vi "BigSky-Sandbox.vi"() -> ()   [LabVIEW 2018]
doc: "This example performs a serial port write and a serial port read. The parameters set for the serial port must match the parameters of the connected instrument or device. The VISA Configure Serial Port VI sets the configuration parameters. The front panel displays the controls used to configure the basic parameters, such as baud rate, data bits, and parity. The VI passes the VISA resource name to other VIs that perform operations on that VISA resource. The VISA Write function sends a command to the serial device and the VISA Read function returns data based on the command. The VISA Close function then closes the reference to the serial device. It is important to close the reference; otherwise, further communication through that port might not be possible."
uses:
  Program Files/National Instruments/LabVIEW 2018/examples/Instrument IO/Serial/support/Serial - Settings.ctl
  <vilib>/Instr/_visa.llb/VISA Configure Serial Port (Instr).vi
panel:
  out "read buffer":string
  in  "write buffer 2":string
  out "Write return count":u32
  in  "byte count":u32=1024
  in  "write buffer":string
  out "Read return count":u32
  in  "Serial Settings":T1={"baud rate"=9600, "data bits"=8, "parity"=enum."None", "stop bits"=10, "flow control"=0} {"flow control" items=["None"=0, "XON/XOFF"=1, "RTS/CTS"=2, "DTR/DSR"=4]; "stop bits" items=["1.0"=10, "1.5"=15, "2.0"=20]; "data bits" min=5 max=8 step=1; "baud rate" items=["75"=75, "110"=110, "134"=134, "150"=150, "300"=300, "600"=600, "1200"=1200, "1800"=1800, "2400"=2400, "4800"=4800, "7200"=7200, "9600"=9600, "14400"=14400, "19200"=19200, "28800"=28800, "38400"=38400, "56000"=56000, "57600"=57600, "115200"=115200, "128000"=128000, "230400"=230400]}
  in  "delay before read (ms)":u32=500
  out "Response":string
  in  "VISA resource name":refnum<visa-resource-name>="COM1"
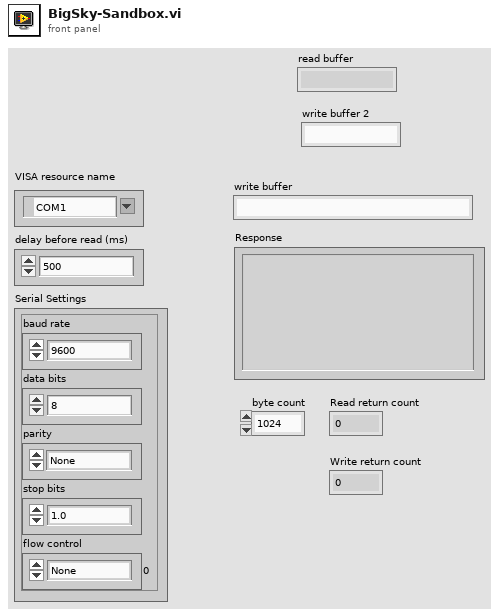
[diagram p1: front panel]
types:
  T1 = typedef "Serial - Settings.ctl" = cluster{"baud rate":u32, "data bits":u16, "parity":enum16{"None", "Odd", "Even", "Mark", "Space"}, "stop bits":u16, "flow control":u16}
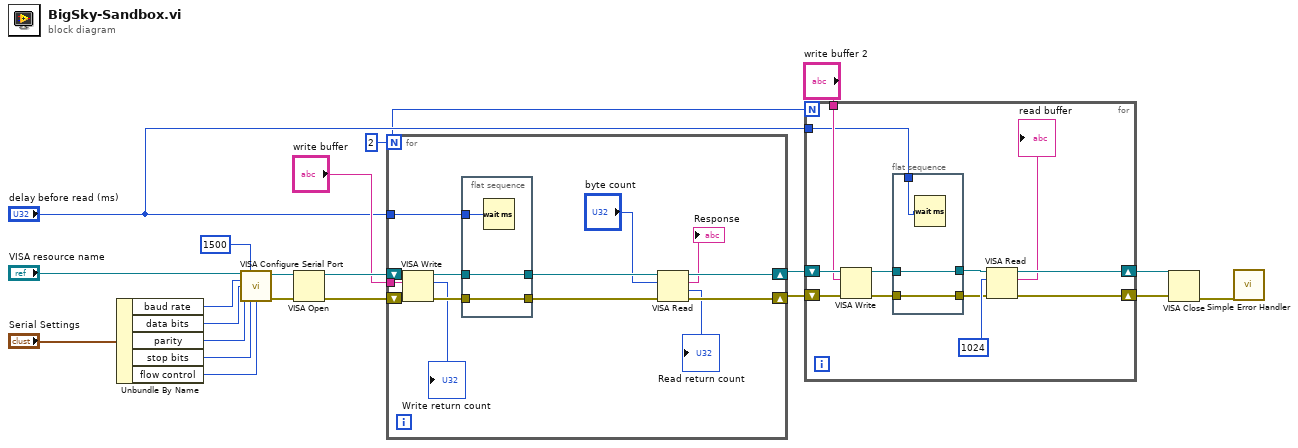
[diagram p0: block diagram]
diagram:
  w1 = 2
  n1 = Unbundle By Name("Serial Settings") -> ("baud rate"=w18:u32, "data bits"=w17:u16, "parity"=w16:enum16{"None", "Odd", "Even", "Mark", "Space"}, "stop bits"=w15:u16, "flow control"=w14:u16)
  n2 = call-poly "VISA Configure Serial Port"("VISA resource name"="VISA resource name", "timeout (10sec)"=u32 1500, "baud rate (9600)"=w18, "data bits (8)"=w17, "parity (0:none)"=w16, "stop bits (10: 1 bit)"=w15, "flow control (0:none)"=w14) -> ("VISA resource name out"=w11:refnum<visa-resource-name>, "error out"=w10:errorcluster)  [unwired: 2 in, 5 out]
  n3 = VISA Open(error in (no error)=w10, VISA resource name=w11) -> (VISA resource name=w13:refnum<visa-resource-name>, error out=w12:errorcluster)  [unwired: 3 in]
  n4 = for {
    N: w1 -> [_]
    tunnel: "delay before read (ms)" -> [w33]
    tunnel: "write buffer" -> [w24]
    shift-right: [w34] -> w5
    shift-left: w13 -> [w32]
    shift-right: [w35] -> w4
    shift-left: w12 -> [w31]
    n5 = VISA Write(VISA resource name=w32, write buffer=w24, error in (no error)=w31) -> (VISA resource name out=w29:refnum<visa-resource-name>, return count=→"Write return count":u32, error out=w30:errorcluster)
    n6 = flat-sequence {
      tunnel: w30 -> [w37]
      tunnel: [w37] -> w26
      tunnel: w29 -> [w36]
      tunnel: [w36] -> w27
      tunnel: w33 -> [w38]
      frame #0 {
        n7 = Wait (ms)(milliseconds to wait=w38) -> ()  [unwired: 1 out]
      }
    }
    n8 = VISA Read(VISA resource name=w27, byte count="byte count", error in (no error)=w26) -> (VISA resource name out=w34:refnum<visa-resource-name>, read buffer=→"Response":string, return count=→"Read return count":u32, error out=w35:errorcluster)
  }
  n9 = for {
    N: w1 -> [_]
    tunnel: "write buffer 2" -> [w46]
    tunnel: "delay before read (ms)" -> [w39]
    shift-right: [w49] -> w6
    shift-left: w5 -> [w48]
    shift-right: [w50] -> w7
    shift-left: w4 -> [w47]
    n10 = VISA Write(VISA resource name=w48, write buffer=w46, error in (no error)=w47) -> (VISA resource name out=w43:refnum<visa-resource-name>, error out=w41:errorcluster)  [unwired: 1 out]
    n11 = flat-sequence {
      tunnel: w43 -> [w53]
      tunnel: [w53] -> w42
      tunnel: w41 -> [w52]
      tunnel: [w52] -> w40
      tunnel: w39 -> [w51]
      frame #0 {
        n12 = Wait (ms)(milliseconds to wait=w51) -> ()  [unwired: 1 out]
      }
    }
    n13 = VISA Read(VISA resource name=w42, byte count=u32 1024, error in (no error)=w40) -> (VISA resource name out=w49:refnum<visa-resource-name>, read buffer=→"read buffer":string, error out=w50:errorcluster)  [unwired: 1 out]
  }
  n14 = VISA Close(VISA resource name=w6, error in (no error)=w7) -> (error out=w20:errorcluster)
  n15 = call <vilib>:"Simple Error Handler.vi"("error in (no error)"=w20) -> ()  [unwired: 1 in, 8 out]
